vi "queryDeviceInterface.vi"(8 "error in (no error)":errorcluster, 11 "IBaseObject in":refnum<class "IBaseObject.lvclass">) -> (0 "error out":errorcluster, 2 "IDevice out":refnum<class "IDevice.lvclass">, 3 "IBaseObject out":refnum<class "IBaseObject.lvclass">)   [LabVIEW 2022 SP3, in "openDAQ.lvlib" / "IBaseObject.lvlib" / "IBaseObject.lvclass"]
uses:
  <instrlib>/openDAQ/Public/Classes/IBaseObject/IBaseObject.lvclass
  <instrlib>/openDAQ/Public/Classes/IBaseObject/IBaseObject.lvclass/IBaseObject.ctl
  <instrlib>/openDAQ/Binaries/Windows/x86/copendaq32.dll
  <instrlib>/openDAQ/Public/Classes/IDevice/IDevice.lvclass
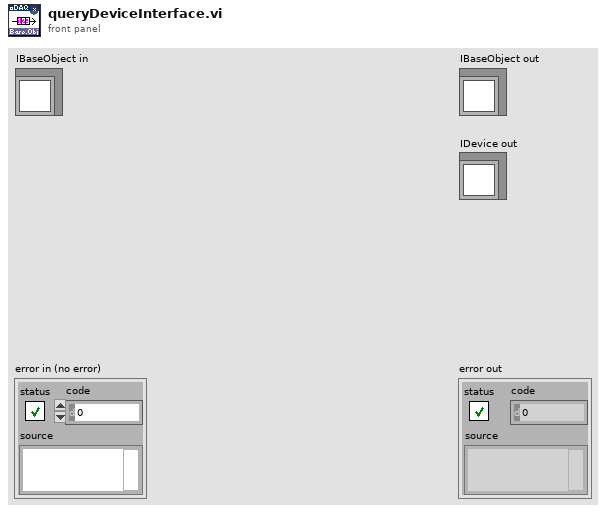
[diagram p1: front panel]
types:
  T1 = enum16{"big-endian, network order", "native, host order", "little-endian"}
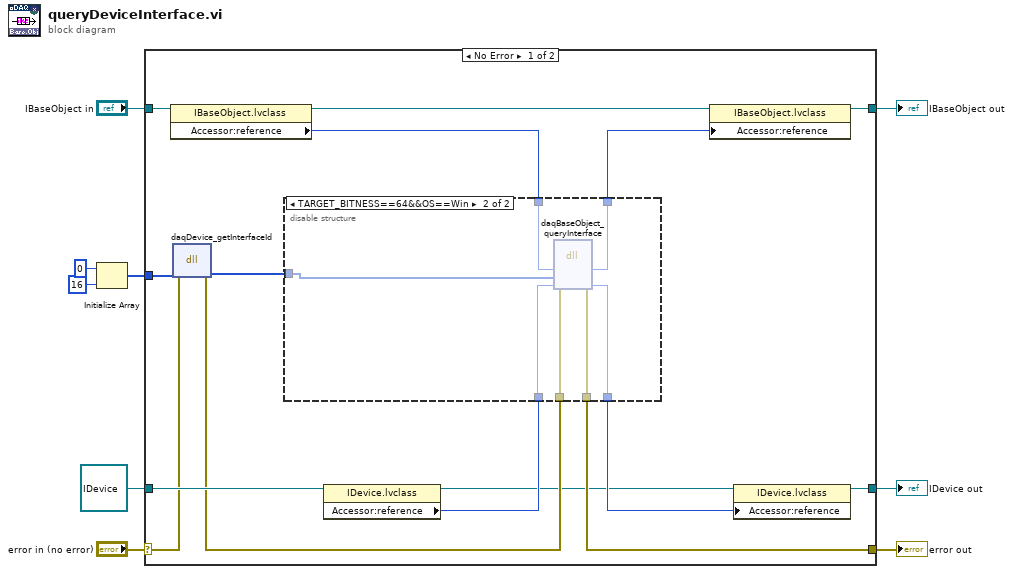
[diagram p0: block diagram]
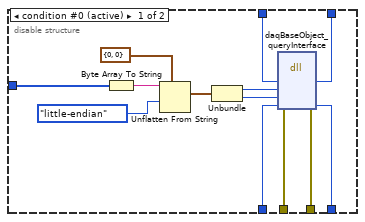
[diagram p2: hidden frame]
diagram:
  n1 = Initialize Array(u8 0, 16 ("dimension size")) -> (w1:u8[])
  n2 = case shown="No Error" "error in (no error)" {
    selector: "error in (no error)" -> [w19 w47]
    tunnel: [w23 w47] -> w8
    tunnel: [w15 w46] -> w6
    tunnel: "IBaseObject in" -> [w24 w46]
    tunnel: refnum<class "IDevice.lvclass"> refnum ("openDAQ.lvlib:IBaseObject.lvlib:IPropertyObject.lvlib:IComponent.lvlib:IFolder.lvlib:IDevice.lvlib:IDevice.lvclass") -> [w22 w45]
    tunnel: w1 -> [w17 _]
    tunnel: [w11 w45] -> w4
    frame No Error {
      n3 = property class="IBaseObject.lvclass"(reference=w24) -> (reference out=w16:refnum<class "IBaseObject.lvclass">, "Accessor:reference"=w21:i64)  [unwired: 1 in, 1 out]
      n4 = dll-call lib="C:/Program Files (x86)/National Instruments/LabVIEW 2022/instr.lib/openDAQ/Binaries/Windows/x86/copendaq*.*" fn="daqDevice_getInterfaceId"(error in=w19, "id"=w17) -> (error out=w18:errorcluster, "id"=w10:u8[])  [unwired: 3 in, 1 out]
      n5 = property class="IDevice.lvclass"(reference=w22) -> (reference out=w12:refnum<class "IDevice.lvclass">, "Accessor:reference"=w20:i64)  [unwired: 1 in, 1 out]
      n6 = disable-structure shown="TARGET_BITNESS==64&&OS==Win" {
        disable-tunnel: [w37 w43] -> w23
        disable-tunnel: w21 -> [w36 w42]
        disable-tunnel: w20 -> [w35 w40]
        disable-tunnel: w18 -> [w34 w44]
        disable-tunnel: [w33 w41] -> w14
        disable-tunnel: [w32 w39] -> w13
        disable-tunnel: w10 -> [w28 w38]
        frame condition #0 (active) {
          n7 = Byte Array To String(unsigned byte array=w28) -> (string=w31:string)
          n8 = Unflatten From String(type=cluster{u64, u64} {0, 0}, binary string=w31, byte order (0:big-endian, network order)=T1."little-endian") -> (value=w29:cluster{u64, u64})  [unwired: 2 in, 2 out]
          n9 = Unbundle(w29) -> (w27:u64, w26:u64)
          n10 = dll-call lib="C:/Program Files (x86)/National Instruments/LabVIEW 2022/instr.lib/openDAQ/Binaries/Windows/x86/copendaq*.*" fn="daqBaseObject_queryInterface"(error in=w34, "self"=w36, "intfId1"=w27, "intfId2"=w26, "interfacePtr"=w35) -> (error out=w37:errorcluster, "self"=w33:i64, "interfacePtr"=w32:i64)  [unwired: 5 in, 1 out]
        }
        frame condition #1 {
          n11 = dll-call lib="C:/Program Files (x86)/National Instruments/LabVIEW 2022/instr.lib/openDAQ/Binaries/Windows/x86/copendaq*.*" fn="daqBaseObject_queryInterface"(error in=w44, "self"=w42, "intfId"=w38, "interfacePtr"=w40) -> (error out=w43:errorcluster, "self"=w41:i64, "interfacePtr"=w39:i64)  [unwired: 4 in, 1 out]
        }
      }
      n12 = property class="IBaseObject.lvclass"(reference=w16, "Accessor:reference"=w14) -> (reference out=w15:refnum<class "IBaseObject.lvclass">)  [unwired: 1 in, 1 out]
      n13 = property class="IDevice.lvclass"(reference=w12, "Accessor:reference"=w13) -> (reference out=w11:refnum<class "IDevice.lvclass">)  [unwired: 1 in, 1 out]
    }
    frame Error {
    }
  }
  "error out" <- w8
  "IBaseObject out" <- w6
  "IDevice out" <- w4
